vi "Get Channel Type.vi"(8 "error in (no error)":errorcluster {"code" format="%.0x"}, 9 "ChannelTypeBufferSize":i32=2048, 10 "Channel":string, 11 "instrument handle":refnum<k15>) -> (0 "error out":errorcluster {"code" format="%.0x"}, 2 "ChannelType":string, 3 "instrument handle out":refnum<k15>)   [LabVIEW 2014, in "Agilent NA.lvlib"]
doc: "Get the type of this channel."
uses:
  Agilent NA.lvlib
  AgNA.dll
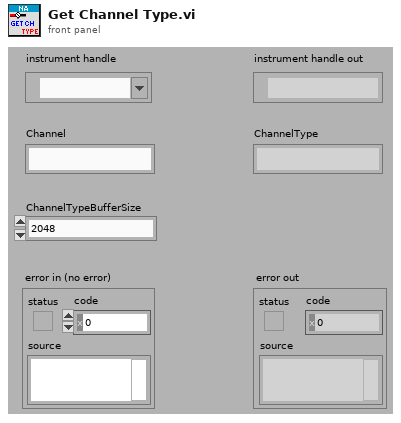
[diagram p1: front panel]
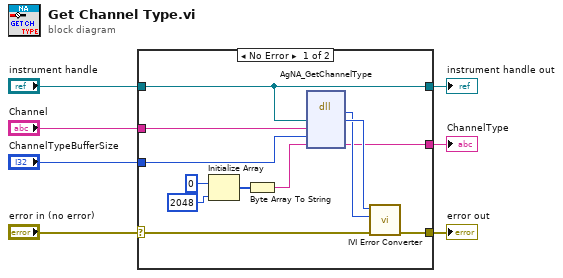
[diagram p0: block diagram]
diagram:
  n1 = case shown="No Error" "error in (no error)" {
    selector: "error in (no error)" -> [w17 w21]
    tunnel: [w16 w21] -> w7
    tunnel: "Channel" -> [w15 _]
    tunnel: "ChannelTypeBufferSize" -> [w14 _]
    tunnel: [w9 _] -> w3
    tunnel: [w8 w20] -> w2
    tunnel: "instrument handle" -> [w8 w20]
    frame No Error {
      n2 = Initialize Array(u8 0 ("element"), 2048 ("dimension size")) -> (w12:u8[])
      n3 = Byte Array To String(unsigned byte array=w12) -> (string=w13:string)
      n4 = dll-call lib="AgNA**.dll" fn="AgNA_GetChannelType"("Vi"=w8, "Channel"=w15, "ChannelTypeBufferSize"=w14, "ChannelType"=w13) -> (w18:i32, "Vi"=w19:u32, "ChannelType"=w9:string)  [unwired: 5 in, 2 out]
      n5 = call "IVI Error Converter.vi"("error in (no error)"=w17, "IVI error code (0)"=w18, "instrument handle"=w19) -> ("error out"=w16:errorcluster)  [unwired: 7 in, 1 out]
    }
    frame Error {
    }
  }
  "error out" <- w7
  "instrument handle out" <- w2
  "ChannelType" <- w3
